vi "Simultaneous Sound Input Output.vi"() -> ()   [LabVIEW 2019]
doc: "This VI illustrates how to perform simultaneous sound IO, i.e., how to continuously play the sound acquired from a microphone. It requires the use of a microphone attached to the sound card. You can specify the IDs of the input and output devices, the frequency to sample at, and the buffer size for both devices. Higher frequencies have better quality, but demand more resources and are limited by the capabilities of your sound card. A large number of samples decreases the risk of glitches, but increases the delay between acquisition and playback."
uses:
  <vilib>/sound2/lvsound2.llb/Sampling Mode.ctl
  <vilib>/sound2/lvsound2.llb/Sound Data Format.ctl
  <vilib>/sound2/lvsound2.llb/Sound Output Write (DBL Single).vi
  <vilib>/sound2/lvsound2.llb/Sound Input Read (DBL).vi
  <vilib>/express/express analysis/Spectral/Block/exnSpectralBlock spectral measurements RMS poly.vi
  <vilib>/express/express analysis/Spectral/Block/exnSpectralBlock spectral measurements RMS WFM.vi
  <vilib>/measure/macond.llb/IIR Filter for 1 Chan.vi
  <vilib>/measure/macond.llb/FIR Filter for 1 Chan.vi
  <vilib>/express/express analysis/Spectral/XNode/ExpressSpectralMeasurementsBlockNode.xnode
  <vilib>/measure/NI_MAPro.lvlib
  <vilib>/measure/NI_MABase.lvlib
panel:
  out "SNR":waveform(dbl)
  out "signal out":waveform(dbl)
  out "FIR filter information":T1={"magnitude H(w)"={"f0"=0.0, "df"=43.06640625, "Mag H(w)"=array[513 elements]}, "phase H(w)"={"f0"=0.0, "df"=43.06640625, "Phase H(w)"=array[513 elements]}, "order"=9}
  out "FIR Frequency Response":cluster{"f0":dbl, "df":dbl, "Mag H(w)":dbl[]}(graph)={"f0"=0.0, "df"=43.06640625, "Mag H(w)"=[-0.019272296926506706, -0.019238324938703828, -0.01913650305983925, -0.018967113472045733, -0.018730626240651423, -0.018427698957270332, -0.018059176241001475, -0.01762608909859478, -0.017129654144702522, -0.016571272683534758, -0.01595252965354438, -0.015275192436914782, -0.014541209535912352, -0.013752709118353258, -0.012911997434660578, -0.012021557109185638, -0.011084045308666909, -0.010102291790903314, -0.009079296836887466, -0.008018229069805418, -0.006922423164506577, -0.00579537745117539, -0.004640751417074567, -0.0034623631103909806, -0.002264186450300432, -0.0010503484475276749, 0.0001748736602943489, 0.0014070553539814509, 0.0026416278543927264, 0.003873881215680502, 0.005098967485521006, 0.006311903927694708, 0.007507576302274881, 0.008680742198692951, 0.009826034416933103, 0.010937964392115054, 0.0120109256577067, 0.013039197342688214, 0.014016947697911862, 0.014938237647088603, 0.0157970243577244, 0.016587164827509732, 0.017302419481656416, 0.017936455776798175, 0.018482851807089914, 0.018935099908328094, 0.01928661025588601, 0.019530714452454717, 0.019660669101675667, 0.019669659363788523, 0.019550802489642565, 0.019297151329445865, 0.018901697812842788, 0.018357376396924353, 0.01765706747906065, 0.016793600771400796, 0.0157597586342061, 0.014548279365153915, 0.013151860442015138, 0.011563161716199758, 0.009774808554756547, 0.007779394928678268, 0.005569486445372527, 0.0031376233234054764, 0.0004763233076461765, -0.0024219154767328396, -0.0055646117330662125, -0.008959298266072968, -0.012613519320165332, -0.01653482798423905, -0.020730783663984436, -0.025208949622576856, -0.02997689059051263, -0.03504217044518283, -0.0404123499607656, -0.0460949846287617, -0.05209762254954174, -0.05842780239505546, -0.06509305144278914, -0.07210088368097765, -0.07945879798497615, -0.0871742763645729, -0.09525478228198339, -0.103707759040182, -0.11254062824109165, -0.12176078831317093, -0.1313756131077903, -0.14139245056376298, -0.15181862143931446, -0.16266141811075058, -0.17392810343697965, -0.1856259096890403, -0.1977620375437153, -0.2103436551402697, -0.22337789719933052, -0.23687186420286746, -0.25083262163422426, -0.265267199277077, -0.2801825905722449, -0.29558575203118653, -0.3114836027050293, -0.32788302370794004, -0.3447908577936766, -0.3622139089840893, -0.3801589422483761, -0.3986326832318677, -0.4176418180331207, -0.437192993028103, -0.45729281474024075, -0.4779478497550988, -0.499164624678501, -0.520949626136852, -0.5433093008184763, -0.5662500555547758, -0.5897782574400124, -0.6139002339885722, -0.6386222733285113, -0.6639506244302827, -0.6898914973694881, -0.716451063622572, -0.7436354563943215, -0.7714507709761588, -0.7999030651341106, -0.8289983595254722, -0.8587426381431261, -0.8891418487865128, -0.92020190355833, -0.9519286793859598, -0.9843280185667381, -1.0174057293361467, -1.051167586458068, -1.085619331836218, -1.120766675145959, -1.1566152944856902, -1.193170837046997, -1.23043891980283, -1.2684251302130067, -1.3071350269462494, -1.3465741406181766, -1.386747974544491, -1.427662005508814, -1.469321684544476, -1.5117324377297505, -1.5548996669959025, -1.5988287509475478, -1.64352504569481, -1.688993885696735, -1.7352405846155619, -1.782270436181323, -1.8300887150664125, -1.8787006777696784, -1.92811156350966, -1.978326595126629, -2.029350979993066, -2.0811899109322636, -2.1338485671447565, -2.1873321151423166, -2.24164570968919, -2.2967944947504333, -2.3527836044470245, -2.4096181640176324, -2.4673032907867984, -2.525844095139398, -2.5852456815012226, -2.6455131493255637, -2.7066515940856584, -2.768666108272939, -2.8315617824009784, -2.895343706015071, -2.9600169687074325, -3.0255866611379574, -3.092057876060508, -3.159435709354809, -3.227725261063878, -3.2969316364370633, -3.367059946978757, -3.4381153115028025, -3.510102857192716, -3.583027720667769, -3.6568950490550813, -3.7317100010678157, -3.807477748089619, -3.884203475265463, -3.961892382599034, -4.040549686056854, -4.120180618679332, -4.200790431698938, -4.28238439566571, -4.364967801580355, -4.448545962035148, -4.5331242123629165, -4.618707911794393, -4.7053024446241585, -4.792913221385569, -4.88154568003489, -4.971205287145045, -5.061897539109232, -5.153627963354877, -5.246402119568165, -5.340225600929644, -5.435104035361241, -5.531043086785116, -5.628048456394799, -5.72612588393903, -5.825281149018785, -5.9255200723979575, -6.026848517328181, -6.129272390888312, -6.2327976453390885, -6.337430279493538, -6.443176340103652, -6.55004192326393, -6.658033175832422, -6.767156296869812, -6.877417539097268, -6.988823210373658, -7.101379675192817, -7.215093356201606, -7.329970735739416, -7.446018357399952, -7.563242827615971, -7.68165081726786, -7.80124906331678, -7.922044370463305, -8.044043612832375, -8.167253735685499, -8.291681757161069, -8.417334770043839, -8.54421994356451, -8.672344525230383, -8.801715842688276, -8.932341305620659, -9.06422840767617, -9.197384728435775, -9.331817935415573, -9.46753578610768, -9.604546130060372, -9.742856910998839, -9.8824761689879, -10.023412042638142, -10.165672771356913, -10.309266697645697, -10.454202269445421, -10.6004880425314, -10.748132682959477, -10.897144969565197, -11.047533796517829, -11.19930817593101, -11.352477240532055, -11.507050246391886, -11.663036575717685, -11.820445739710442, -11.979287381489584, -12.139571279087129, -12.301307348513626, -12.464505646898537, -12.629176375707585, -12.795329884039756, -12.962976672006866, -13.132127394198479, -13.302792863235355, -13.474984053414476, -13.648712104448997, -13.82398832530651, -14.000824198149232, -14.17923138237975, -14.359221718796247, -14.5408072338612, -14.724000144087722, -14.908812860547977, -15.095257993508156, -15.283348357194814, -15.47309697469746, -15.664517083012658, -15.85762213823501, -16.052425820900563, -16.248942041488704, -16.447184946088573, -16.64716892223645, -16.848908604930905, -17.052418882832665, -17.257714904656677, -17.464812085763892, -17.673726114961102, -17.88447296151708, -18.097068882403946, -18.311530429773132, -18.52787445867555, -18.746118135036344, -18.966278943894817, -19.18837469792084, -19.412423546219692, -19.638443983437565, -19.866454859180916, -20.096475387763455, -20.328525158295076, -20.562624145128048, -20.7987927186766, -21.037051656626353, -21.277422155551978, -21.519925842961317, -21.764584789786024, -22.011421523339436, -22.26045904076386, -22.511720822990327, -22.765230849235664, -23.021013612062617, -23.2790941330307, -23.539497978966786, -23.80225127888623, -24.067380741597315, -24.334913674023415, -24.604878000279648, -24.877302281543102, -25.15221573675766, -25.429648264217736, -25.709630464077225, -25.992193661833557, -26.277369932839655, -26.565192127900037, -26.855693900010937, -27.14890973230865, -27.444874967293842, -27.743625837405204, -28.04519949701978, -28.34963405596346, -28.65696861462039, -28.967243300736726, -29.280499308020737, -29.596778936648796, -29.91612563579445, -30.23858404830711, -30.564200057675283, -30.893020837420924, -31.22509490308107, -31.56047216694642, -31.89920399573895, -32.24134327142523, -32.58694445537889, -32.93606365612077, -33.28875870088696, -33.645089211293715, -34.00511668339162, -34.368904572427, -34.73651838265499, -35.108025762580255, -35.483496606033526, -35.863003159530955, -36.246620136401994, -36.634424838218244, -37.02649728410583, -37.422920348579005, -37.82377990859529, -38.22916500060143, -38.63916798841565, -39.05388474288023, -39.473414834311384, -39.89786173888482, -40.327333060213505, -40.761940767515206, -41.201801451915124, -41.64703660261034, -42.097772904810626, -42.55414256160428, -43.01628364213889, -43.48434045880812, -43.95846397645467, -44.43881225698491, -44.92555094321597, -45.4188537862839, -45.91890322150131, -46.42589099823071, -46.94001887009429, -47.461499352747325, -47.99055655747627, -48.52742711010177, -49.07236116610441, -49.625623534568945, -50.18749492553697, -50.75827333772171, -51.33827560635321, -51.927839134282685, -52.5273238335194, -53.13711430924978, -53.757622324287986, -54.38928958910903, -55.03259093141922, -55.68803791006044, -56.356182951456475, -57.03762410353738, -57.73301052300722, -58.443048838265256, -59.168510563887516, -59.910240785594425, -60.669168390196255, -61.44631818735503, -62.242825365125036, -63.05995284747673, -63.899112291461606, -64.76188969162212, -65.65007687529862, -66.56571061263774, -67.51112168728602, -68.48899716720864, -69.5024604209681, -70.55517537064686, -71.651484434526, -72.79659423077602, -73.99683050792132, -75.25999597273162, -76.59588553683317, -78.01705056824085, -79.53997274478137, -81.18694382708803, -82.98923275619033, -84.99277082433886, -87.26922420262144, -89.94005397741844, -93.23764235650287, -97.70409035926502, -105.2389549546036, -120.21940212694396, -103.87434379024525, -99.25657740918373, -96.75346852480884, -95.19229210275768, -94.1769311801686, -93.52621522867429, -93.14331610943202, -92.97170063781878, -92.9769036052985, -93.13798339386565, -93.44324991006425, -93.88817300465095, -94.47461965509477, -95.21114046171355, -96.11440828293355, -97.21236213863213, -98.55046167774603, -100.20455346957709, -102.31005945327479, -105.13999077012153, -109.38026102744627, -117.90316417153689, -121.74968794633244, -110.87465769391795, -106.30673031397427, -103.4257036819042, -101.35345183307467, -99.76224656663788, -98.4932397160122, -97.45718163832082, -96.59885132300386, -95.88167048439843, -95.28014683386081, -94.77580353423141, -94.35482631386327, -94.00662541854528, -93.72291598478472, -93.4971074631025, -93.32388523212437, -93.19891609508849, -93.1186361322281, -93.080094793469, -93.08083832038712, -93.11882125722646, -93.19233841023629, -93.29997195218314, -93.44054992699938, -93.61311346463015, -93.816890746238, -94.05127627467188, -94.31581437091336, -94.61018608389674, -94.93419889552317, -95.2877787487493, -95.6709640354363, -96.08390126254123, -96.5268421810798, -97.00014220905646, -97.50426001733464, -98.03975817855428, -98.60730479719669, -99.20767605815145, -99.84175963718543, -100.51055892552911, -101.21519801731345, -101.9569274076452, -102.73713033893578, -103.5573297268468, -104.41919559235856, -105.32455293724834, -106.27539004452969, -107.2738673041816, -108.32232691557408, -109.42330434606752, -110.57954342631754, -111.79401886908653, -113.0699735210075, -114.41098407326743, -115.82108070934652, -117.30496747515284, -118.86842927370196, -120.51908410052798, -122.26777819390442, -124.13120028023899, -126.13689088843186, -128.33325735095758, -130.8111634602009, -133.7568780642302, -137.61413678937367, -143.8430103069744, -inf]}
  out "IIR filter information":T1={"magnitude H(w)"={"f0"=0.0, "df"=43.06640625, "Mag H(w)"=array[513 elements]}, "phase H(w)"={"f0"=0.0, "df"=43.06640625, "Phase H(w)"=array[513 elements]}, "order"=9}
  in  "Tab Control":T2(tab)=enum."IIR"
  out "Waveform Graph":cluster{"f0":dbl, "df":dbl, "magnitude":dbl[]}(graph)
  in  "IIR filter specifications":T3={"Topology"=enum."Butterworth", "Type"=enum."Lowpass", "Order"=4, "Lower Fc"=2000.0, "Upper Fc"=200.0, "PB Ripple"=1.0, "SB Attenuation"=60.0} {"PB Ripple" format="%0.2f"; "SB Attenuation" format="%0.2f"; "Lower Fc" format="%0.2p"; "Upper Fc" format="%0.2p"}
  in  "FIR filter specifications":T4={"Topology"=enum."FIR by Specification", "Type"=enum."Lowpass", "#Taps"=10, "Lower PB"=3000.0, "Upper PB"=0.0, "Lower SB"=18000.0, "Upper SB"=0.0} {"Lower SB" format="%0.2p"; "Upper SB" format="%0.2p"; "Lower PB" format="%0.2p"; "Upper PB" format="%0.2p"}
  in  "optional FIR filter specifications":T5={"PB Gain"=0.00868, "SB Gain"=-100.0, "Scale"=TRUE, "Window"=enum."Flat Top"} {"SB Gain" format="%.2p"; "PB Gain" format="%.2p"}
  in  "standard deviation":dbl=1.0 format="%.2p"
  out "IIR Frequency Response":cluster{"f0":dbl, "df":dbl, "Mag H(w)":dbl[]}(graph)={"f0"=0.0, "df"=43.06640625, "Mag H(w)"=[-0.019272296926506706, -0.019238324938703828, -0.01913650305983925, -0.018967113472045733, -0.018730626240651423, -0.018427698957270332, -0.018059176241001475, -0.01762608909859478, -0.017129654144702522, -0.016571272683534758, -0.01595252965354438, -0.015275192436914782, -0.014541209535912352, -0.013752709118353258, -0.012911997434660578, -0.012021557109185638, -0.011084045308666909, -0.010102291790903314, -0.009079296836887466, -0.008018229069805418, -0.006922423164506577, -0.00579537745117539, -0.004640751417074567, -0.0034623631103909806, -0.002264186450300432, -0.0010503484475276749, 0.0001748736602943489, 0.0014070553539814509, 0.0026416278543927264, 0.003873881215680502, 0.005098967485521006, 0.006311903927694708, 0.007507576302274881, 0.008680742198692951, 0.009826034416933103, 0.010937964392115054, 0.0120109256577067, 0.013039197342688214, 0.014016947697911862, 0.014938237647088603, 0.0157970243577244, 0.016587164827509732, 0.017302419481656416, 0.017936455776798175, 0.018482851807089914, 0.018935099908328094, 0.01928661025588601, 0.019530714452454717, 0.019660669101675667, 0.019669659363788523, 0.019550802489642565, 0.019297151329445865, 0.018901697812842788, 0.018357376396924353, 0.01765706747906065, 0.016793600771400796, 0.0157597586342061, 0.014548279365153915, 0.013151860442015138, 0.011563161716199758, 0.009774808554756547, 0.007779394928678268, 0.005569486445372527, 0.0031376233234054764, 0.0004763233076461765, -0.0024219154767328396, -0.0055646117330662125, -0.008959298266072968, -0.012613519320165332, -0.01653482798423905, -0.020730783663984436, -0.025208949622576856, -0.02997689059051263, -0.03504217044518283, -0.0404123499607656, -0.0460949846287617, -0.05209762254954174, -0.05842780239505546, -0.06509305144278914, -0.07210088368097765, -0.07945879798497615, -0.0871742763645729, -0.09525478228198339, -0.103707759040182, -0.11254062824109165, -0.12176078831317093, -0.1313756131077903, -0.14139245056376298, -0.15181862143931446, -0.16266141811075058, -0.17392810343697965, -0.1856259096890403, -0.1977620375437153, -0.2103436551402697, -0.22337789719933052, -0.23687186420286746, -0.25083262163422426, -0.265267199277077, -0.2801825905722449, -0.29558575203118653, -0.3114836027050293, -0.32788302370794004, -0.3447908577936766, -0.3622139089840893, -0.3801589422483761, -0.3986326832318677, -0.4176418180331207, -0.437192993028103, -0.45729281474024075, -0.4779478497550988, -0.499164624678501, -0.520949626136852, -0.5433093008184763, -0.5662500555547758, -0.5897782574400124, -0.6139002339885722, -0.6386222733285113, -0.6639506244302827, -0.6898914973694881, -0.716451063622572, -0.7436354563943215, -0.7714507709761588, -0.7999030651341106, -0.8289983595254722, -0.8587426381431261, -0.8891418487865128, -0.92020190355833, -0.9519286793859598, -0.9843280185667381, -1.0174057293361467, -1.051167586458068, -1.085619331836218, -1.120766675145959, -1.1566152944856902, -1.193170837046997, -1.23043891980283, -1.2684251302130067, -1.3071350269462494, -1.3465741406181766, -1.386747974544491, -1.427662005508814, -1.469321684544476, -1.5117324377297505, -1.5548996669959025, -1.5988287509475478, -1.64352504569481, -1.688993885696735, -1.7352405846155619, -1.782270436181323, -1.8300887150664125, -1.8787006777696784, -1.92811156350966, -1.978326595126629, -2.029350979993066, -2.0811899109322636, -2.1338485671447565, -2.1873321151423166, -2.24164570968919, -2.2967944947504333, -2.3527836044470245, -2.4096181640176324, -2.4673032907867984, -2.525844095139398, -2.5852456815012226, -2.6455131493255637, -2.7066515940856584, -2.768666108272939, -2.8315617824009784, -2.895343706015071, -2.9600169687074325, -3.0255866611379574, -3.092057876060508, -3.159435709354809, -3.227725261063878, -3.2969316364370633, -3.367059946978757, -3.4381153115028025, -3.510102857192716, -3.583027720667769, -3.6568950490550813, -3.7317100010678157, -3.807477748089619, -3.884203475265463, -3.961892382599034, -4.040549686056854, -4.120180618679332, -4.200790431698938, -4.28238439566571, -4.364967801580355, -4.448545962035148, -4.5331242123629165, -4.618707911794393, -4.7053024446241585, -4.792913221385569, -4.88154568003489, -4.971205287145045, -5.061897539109232, -5.153627963354877, -5.246402119568165, -5.340225600929644, -5.435104035361241, -5.531043086785116, -5.628048456394799, -5.72612588393903, -5.825281149018785, -5.9255200723979575, -6.026848517328181, -6.129272390888312, -6.2327976453390885, -6.337430279493538, -6.443176340103652, -6.55004192326393, -6.658033175832422, -6.767156296869812, -6.877417539097268, -6.988823210373658, -7.101379675192817, -7.215093356201606, -7.329970735739416, -7.446018357399952, -7.563242827615971, -7.68165081726786, -7.80124906331678, -7.922044370463305, -8.044043612832375, -8.167253735685499, -8.291681757161069, -8.417334770043839, -8.54421994356451, -8.672344525230383, -8.801715842688276, -8.932341305620659, -9.06422840767617, -9.197384728435775, -9.331817935415573, -9.46753578610768, -9.604546130060372, -9.742856910998839, -9.8824761689879, -10.023412042638142, -10.165672771356913, -10.309266697645697, -10.454202269445421, -10.6004880425314, -10.748132682959477, -10.897144969565197, -11.047533796517829, -11.19930817593101, -11.352477240532055, -11.507050246391886, -11.663036575717685, -11.820445739710442, -11.979287381489584, -12.139571279087129, -12.301307348513626, -12.464505646898537, -12.629176375707585, -12.795329884039756, -12.962976672006866, -13.132127394198479, -13.302792863235355, -13.474984053414476, -13.648712104448997, -13.82398832530651, -14.000824198149232, -14.17923138237975, -14.359221718796247, -14.5408072338612, -14.724000144087722, -14.908812860547977, -15.095257993508156, -15.283348357194814, -15.47309697469746, -15.664517083012658, -15.85762213823501, -16.052425820900563, -16.248942041488704, -16.447184946088573, -16.64716892223645, -16.848908604930905, -17.052418882832665, -17.257714904656677, -17.464812085763892, -17.673726114961102, -17.88447296151708, -18.097068882403946, -18.311530429773132, -18.52787445867555, -18.746118135036344, -18.966278943894817, -19.18837469792084, -19.412423546219692, -19.638443983437565, -19.866454859180916, -20.096475387763455, -20.328525158295076, -20.562624145128048, -20.7987927186766, -21.037051656626353, -21.277422155551978, -21.519925842961317, -21.764584789786024, -22.011421523339436, -22.26045904076386, -22.511720822990327, -22.765230849235664, -23.021013612062617, -23.2790941330307, -23.539497978966786, -23.80225127888623, -24.067380741597315, -24.334913674023415, -24.604878000279648, -24.877302281543102, -25.15221573675766, -25.429648264217736, -25.709630464077225, -25.992193661833557, -26.277369932839655, -26.565192127900037, -26.855693900010937, -27.14890973230865, -27.444874967293842, -27.743625837405204, -28.04519949701978, -28.34963405596346, -28.65696861462039, -28.967243300736726, -29.280499308020737, -29.596778936648796, -29.91612563579445, -30.23858404830711, -30.564200057675283, -30.893020837420924, -31.22509490308107, -31.56047216694642, -31.89920399573895, -32.24134327142523, -32.58694445537889, -32.93606365612077, -33.28875870088696, -33.645089211293715, -34.00511668339162, -34.368904572427, -34.73651838265499, -35.108025762580255, -35.483496606033526, -35.863003159530955, -36.246620136401994, -36.634424838218244, -37.02649728410583, -37.422920348579005, -37.82377990859529, -38.22916500060143, -38.63916798841565, -39.05388474288023, -39.473414834311384, -39.89786173888482, -40.327333060213505, -40.761940767515206, -41.201801451915124, -41.64703660261034, -42.097772904810626, -42.55414256160428, -43.01628364213889, -43.48434045880812, -43.95846397645467, -44.43881225698491, -44.92555094321597, -45.4188537862839, -45.91890322150131, -46.42589099823071, -46.94001887009429, -47.461499352747325, -47.99055655747627, -48.52742711010177, -49.07236116610441, -49.625623534568945, -50.18749492553697, -50.75827333772171, -51.33827560635321, -51.927839134282685, -52.5273238335194, -53.13711430924978, -53.757622324287986, -54.38928958910903, -55.03259093141922, -55.68803791006044, -56.356182951456475, -57.03762410353738, -57.73301052300722, -58.443048838265256, -59.168510563887516, -59.910240785594425, -60.669168390196255, -61.44631818735503, -62.242825365125036, -63.05995284747673, -63.899112291461606, -64.76188969162212, -65.65007687529862, -66.56571061263774, -67.51112168728602, -68.48899716720864, -69.5024604209681, -70.55517537064686, -71.651484434526, -72.79659423077602, -73.99683050792132, -75.25999597273162, -76.59588553683317, -78.01705056824085, -79.53997274478137, -81.18694382708803, -82.98923275619033, -84.99277082433886, -87.26922420262144, -89.94005397741844, -93.23764235650287, -97.70409035926502, -105.2389549546036, -120.21940212694396, -103.87434379024525, -99.25657740918373, -96.75346852480884, -95.19229210275768, -94.1769311801686, -93.52621522867429, -93.14331610943202, -92.97170063781878, -92.9769036052985, -93.13798339386565, -93.44324991006425, -93.88817300465095, -94.47461965509477, -95.21114046171355, -96.11440828293355, -97.21236213863213, -98.55046167774603, -100.20455346957709, -102.31005945327479, -105.13999077012153, -109.38026102744627, -117.90316417153689, -121.74968794633244, -110.87465769391795, -106.30673031397427, -103.4257036819042, -101.35345183307467, -99.76224656663788, -98.4932397160122, -97.45718163832082, -96.59885132300386, -95.88167048439843, -95.28014683386081, -94.77580353423141, -94.35482631386327, -94.00662541854528, -93.72291598478472, -93.4971074631025, -93.32388523212437, -93.19891609508849, -93.1186361322281, -93.080094793469, -93.08083832038712, -93.11882125722646, -93.19233841023629, -93.29997195218314, -93.44054992699938, -93.61311346463015, -93.816890746238, -94.05127627467188, -94.31581437091336, -94.61018608389674, -94.93419889552317, -95.2877787487493, -95.6709640354363, -96.08390126254123, -96.5268421810798, -97.00014220905646, -97.50426001733464, -98.03975817855428, -98.60730479719669, -99.20767605815145, -99.84175963718543, -100.51055892552911, -101.21519801731345, -101.9569274076452, -102.73713033893578, -103.5573297268468, -104.41919559235856, -105.32455293724834, -106.27539004452969, -107.2738673041816, -108.32232691557408, -109.42330434606752, -110.57954342631754, -111.79401886908653, -113.0699735210075, -114.41098407326743, -115.82108070934652, -117.30496747515284, -118.86842927370196, -120.51908410052798, -122.26777819390442, -124.13120028023899, -126.13689088843186, -128.33325735095758, -130.8111634602009, -133.7568780642302, -137.61413678937367, -143.8430103069744, -inf]}
  out "Acquired Sound":waveform(dbl)(graph)={"t0"=timestamp(3727379422.426577 s since 1904-01-01), "dt"=2.2675736961451248e-05, "Y"=array[10000 elements]}
  in  "Stop":bool
  in  "Input Device ID":u32=2
  in  "Output Device ID":u32=2
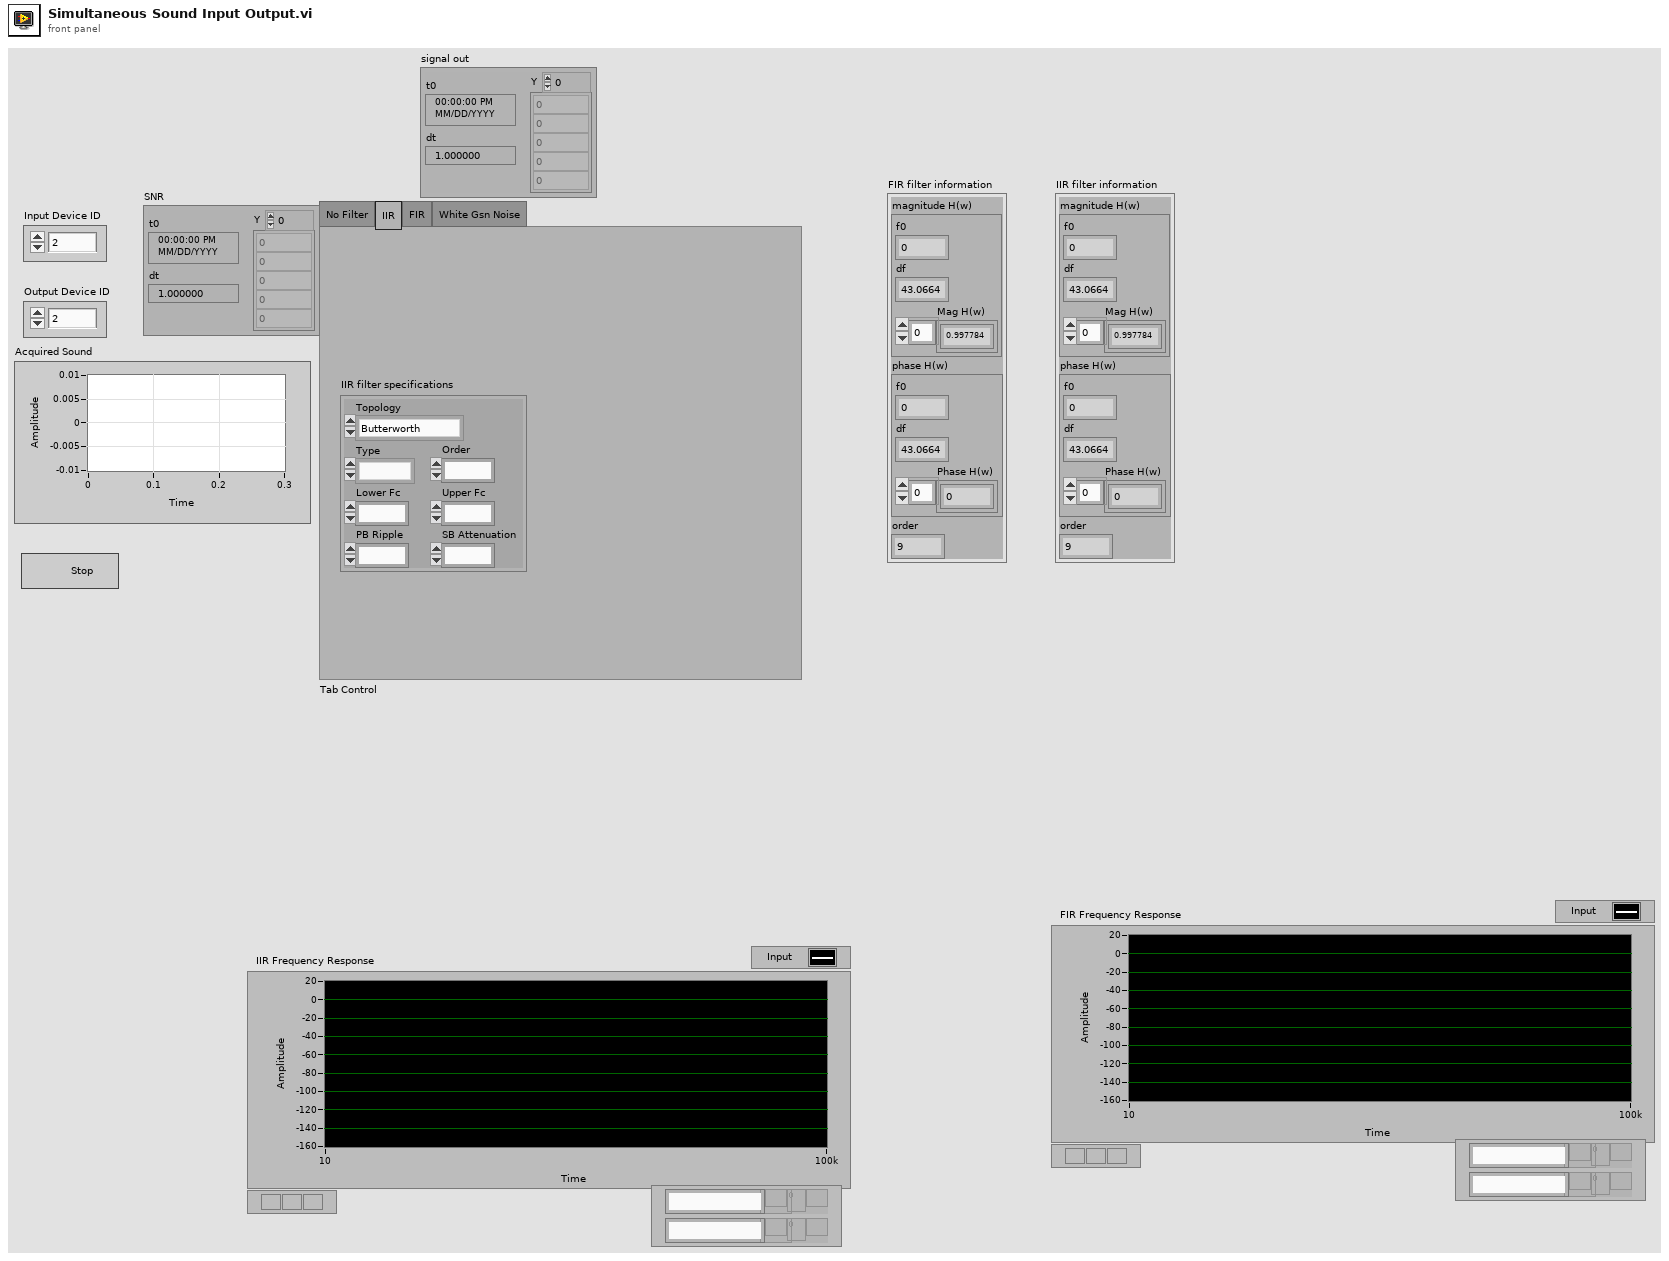
[diagram p1: front panel]
types:
  T1 = cluster{"magnitude H(w)":cluster{"f0":dbl, "df":dbl, "Mag H(w)":dbl[]}, "phase H(w)":cluster{"f0":dbl, "df":dbl, "Phase H(w)":dbl[]}, "order":i32}
  T2 = enum32{"No Filter", "IIR", "FIR", "White Gsn Noise"}
  T3 = cluster{"Topology":enum16{"Off", "Butterworth", "Chebyshev", "Inverse Chebyshev", "Elliptic", "Bessel"}, "Type":enum16{"Lowpass", "Highpass", "Bandpass", "Bandstop"}, "Order":i32, "Lower Fc":dbl, "Upper Fc":dbl, "PB Ripple":dbl, "SB Attenuation":dbl}
  T4 = cluster{"Topology":enum16{"Off", "FIR by Specification", "Equi-ripple FIR", "Windowed FIR"}, "Type":enum16{"Lowpass", "Highpass", "Bandpass", "Bandstop"}, "#Taps":i32, "Lower PB":dbl, "Upper PB":dbl, "Lower SB":dbl, "Upper SB":dbl}
  T5 = cluster{"PB Gain":dbl, "SB Gain":dbl, "Scale":bool, "Window":enum16{"None", "Hanning", "Hamming", "Triangular", "Blackman", "Exact Blackman", "Blackman-Harris", "Kaiser-Bessel", "Flat Top"}}
  T6 = typedef "Sound Data Format.ctl" = cluster{"sample rate (S/s)":dbl, "number of channels":i32, "bits per sample":i32}
  T7 = typedef "Sampling Mode.ctl" = i32
  T8 = typedef "Sound Output Task ID.ctl" = u32
  T9 = typedef "Sound Input Task ID.ctl" = u32
  T10 = cluster{"averaging mode":u16, "weighting mode":u16, "number of averages":u32}
  T11 = cluster{"dB On (F)":bool, "unwrap phase (F)":bool, "convert to degree (F)":bool}
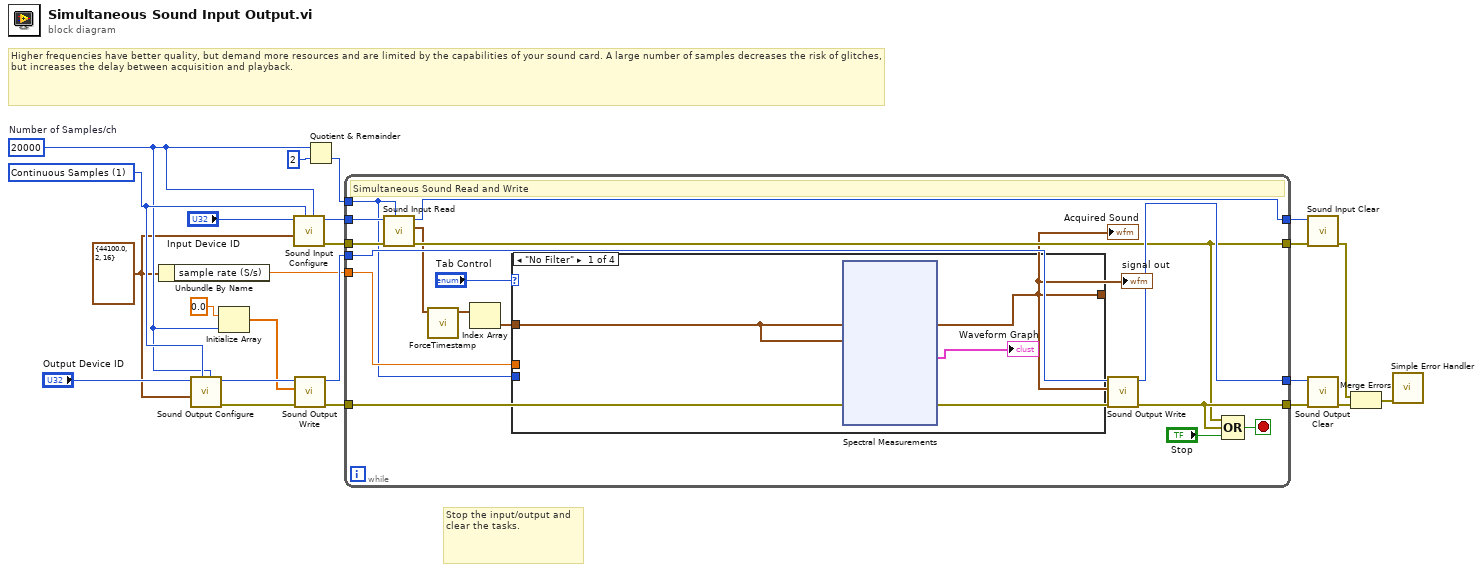
[diagram p0: block diagram]
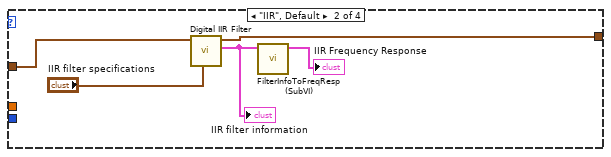
[diagram p2: hidden frame]
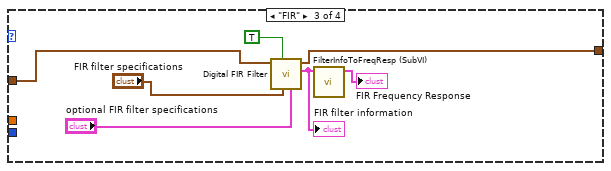
[diagram p3: hidden frame]
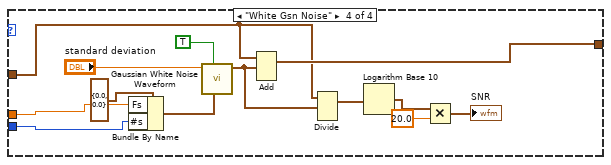
[diagram p4: hidden frame]
diagram:
  w4 = 20000  # Number of Samples/ch
  w2 = T6 {"sample rate (S/s)"=44100.0, "number of channels"=2, "bits per sample"=16} ("Sound Format")
  w13 = T7 1 items=["Finite Samples", "Continuous Samples"] ("sample mode")
  # "Higher frequencies have better quality, but demand more resources and are limited by the capabilities of your sound card. A large number of samples decreases the risk of glitches, but increases the delay between acquisition and playback."
  # "Stop the input/output and clear the tasks."
  n1 = Unbundle By Name(w2) -> ("sample rate (S/s)"=w1:dbl)
  n2 = call <vilib>:"Sound Output Configure.vi"("number of samples/ch"=w4, "sample mode"=w13, "sound format"=w2, "device ID"="Output Device ID") -> ("error out"=w11:errorcluster, "task ID"=w12:T8)  [unwired: 6 in]
  n3 = Initialize Array(0.0 ("element"), w4) -> (w6:dbl[])
  n4 = call <vilib>:"Sound Input Configure.vi"("number of samples/ch"=w4, "sample mode"=w13, "sound format"=w2, "device ID"="Input Device ID") -> ("error out"=w15:errorcluster, "task ID"=w14:T9)  [unwired: 6 in]
  n5 = call-poly <vilib>:"Sound Output Write.vi"("error in (no error)"=w11, "data"=w6, "task ID"=w12) -> ("error out"=w10:errorcluster, "task ID out"=w9:T8)  [unwired: 7 in]
  n6 = Quotient & Remainder(x=w4, y=2) -> (floor(x/y)=w5:i32)  [unwired: 1 out]
  n7 = while {
    tunnel: w5 -> [w25]
    tunnel: w14 -> [w38]
    tunnel: [w36] -> w18
    tunnel: w9 -> [w39]
    tunnel: [w37] -> w21
    tunnel: w10 -> [w35]
    tunnel: [w32] -> w22
    tunnel: w15 -> [w40]
    tunnel: [w31] -> w23
    tunnel: w1 -> [w26]
    stop <- w33 stop-if-true
    # "Simultaneous Sound Read and Write"
    n8 = call-poly <vilib>:"Sound Input Read.vi"("number of samples/ch"=w25, "error in (no error)"=w40, "task ID"=w38) -> ("error out"=w31:errorcluster, "data"=w30:waveform(dbl)[], "task ID out"=w36:T9)  [unwired: 6 in]
    n9 = call "ForceTimestamp.vi"("In"=w30) -> ("Out"=w29:waveform(dbl)[])  [unwired: 10 in]
    n10 = Index Array(array=w29) -> (element=w27:waveform(dbl))  [unwired: 1 in]
    n11 = case shown="\"No Filter\"" "Tab Control" {
      tunnel: w27 -> [w42 w57 w61 w70]
      tunnel: [w42 w55 w60 w75] -> w24
      tunnel: w26 -> [_ _ _ w72]
      tunnel: w25 -> [_ _ _ w71]
      frame "No Filter" {
        n12 = xnode "Spectral Measurements"("Signals"=w42) -> ("FFT - (RMS)"=→"Waveform Graph":cluster{"f0":dbl, "df":dbl, "magnitude":dbl[]})  [unwired: 1 in, 2 out]
      }
      frame "IIR", Default {
        n13 = call-poly <vilib>:"Digital IIR Filter.vi"("IIR filter specifications"="IIR filter specifications", "signal in"=w57) -> ("filter information"=w53:T1, "signal out"=w55:waveform(dbl))  [unwired: 7 in, 1 out]
        "IIR filter information" <- w53
        n14 = call "FilterInfoToFreqResp (SubVI).vi"("filter information"=w53) -> ("Frequency Response"=→"IIR Frequency Response":cluster{"f0":dbl, "df":dbl, "Mag H(w)":dbl[]})  [unwired: 10 in]
      }
      frame "FIR" {
        n15 = call-poly <vilib>:"Digital FIR Filter.vi"("optional FIR filter specifications"="optional FIR filter specifications", "FIR filter specifications"="FIR filter specifications", "reset filter"=TRUE, "signal in"=w61) -> ("filter information"=w58:T1, "signal out"=w60:waveform(dbl))  [unwired: 5 in, 1 out]
        "FIR filter information" <- w58
        n16 = call "FilterInfoToFreqResp (SubVI).vi"("filter information"=w58) -> ("Frequency Response"=→"FIR Frequency Response":cluster{"f0":dbl, "df":dbl, "Mag H(w)":dbl[]})  [unwired: 10 in]
      }
      frame "White Gsn Noise" {
        n17 = Bundle By Name(cluster=cluster{"Fs":dbl, "#s":dbl} {"Fs"=0.0, "#s"=0.0} ("sampling info"), "Fs"=w72, "#s"=w71) -> (w73:cluster{"Fs":dbl, "#s":dbl})
        n18 = call <vilib>:"Gaussian White Noise Waveform.vi"("sampling info"=w73, "reset signal"=TRUE, "standard deviation"="standard deviation") -> ("signal out"=w69:waveform(dbl))  [unwired: 7 in, 1 out]
        n19 = Add(1:w69, 2:w70) -> (0:w75:waveform(dbl))  [unwired: 1 in, 1 out]
        n20 = Divide(1:w69, 2:w70) -> (0:w68:waveform(dbl))  [unwired: 1 in, 1 out]
        n21 = Logarithm Base 10(1:w68) -> (0:w67:waveform(dbl))
        n22 = Multiply(x=w67, y=20.0) -> (x*y=→"SNR":waveform(dbl))
      }
    }
    "Acquired Sound" <- w24
    "signal out" <- w24
    n23 = call-poly <vilib>:"Sound Output Write.vi"("error in (no error)"=w35, "data"=w24, "task ID"=w39) -> ("error out"=w32:errorcluster, "task ID out"=w37:T8)  [unwired: 7 in]
    n24 = Compound Arithmetic op=OR(w31, w32, "Stop") -> (w33:bool)
  }
  n25 = call <vilib>:"Sound Input Clear.vi"("error in (no error)"=w23, "task ID"=w18) -> ("error out"=w16:errorcluster)  [unwired: 9 in]
  n26 = call <vilib>:"Sound Output Clear.vi"("error in (no error)"=w22, "task ID"=w21) -> ("error out"=w17:errorcluster)  [unwired: 9 in]
  n27 = Merge Errors(w16, w17) -> (w8:errorcluster)
  n28 = call <vilib>:"Simple Error Handler.vi"("error in (no error)"=w8) -> ()  [unwired: 4 in, 5 out]
